vi "Write StartRX.vi"(8 "error in (no error)":errorcluster, 10 "StartRX":refnum<k24>, 11 "HRF_Device in":refnum<class "HRF_Device.lvclass">) -> (0 "error out":errorcluster, 3 "HRF_Device out":refnum<class "HRF_Device.lvclass">)   [LabVIEW 2020, in "HRF_Device.lvclass"]
uses:
  HRF_Device.lvclass
  D:/work/HackRF/Labview Driver/NetHackrf.dll
  NetHackrf.dll
  HRF_Device.lvclass/HRF_Device.ctl
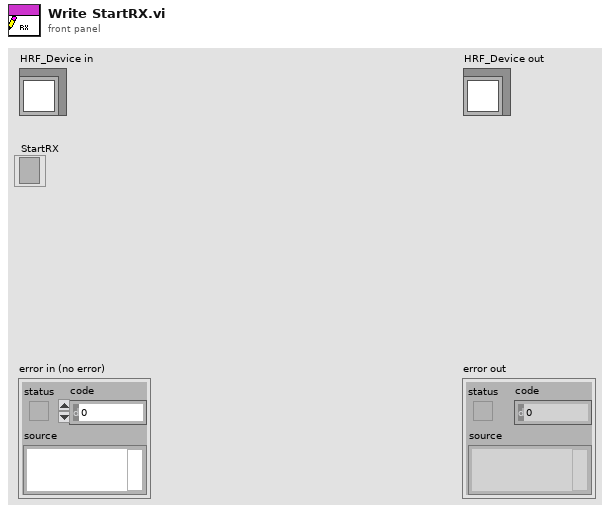
[diagram p1: front panel]
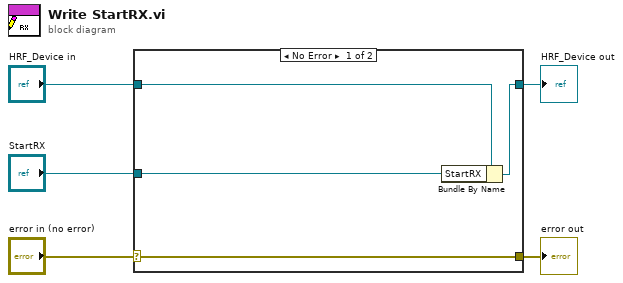
[diagram p0: block diagram]
diagram:
  n1 = case shown="No Error" "error in (no error)" {
    selector: "error in (no error)" -> [w9 w10]
    tunnel: [w9 w10] -> w4
    tunnel: [w7 w11] -> w2
    tunnel: "HRF_Device in" -> [w8 w11]
    tunnel: "StartRX" -> [w6 _]
    frame No Error {
      n2 = Bundle By Name(cluster=w8, "StartRX"=w6) -> (w7:refnum<class "HRF_Device.lvclass">)
    }
    frame Error {
    }
  }
  "error out" <- w4
  "HRF_Device out" <- w2
